vi "LoadFiles.vi"   [LabVIEW 2014]
uses:
  Common Code/Change Detect Int.vi
  Robot Global Data.vi
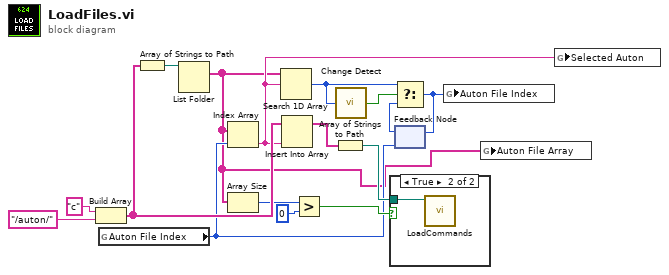
[diagram p0: block diagram]
diagram:
  n1 = Build Array("c", "/auton/") -> (w13:string[])
  n2 = global read "Robot Global Data.vi" "Auton File Index"() -> (w4:i32)
  n3 = Array of Strings to Path(0:w13) -> (2:w14:path)  [unwired: 1 in]
  n4 = List Folder(path=w14) -> (filenames=w1:string[])  [unwired: 3 in, 3 out]
  n5 = Index Array(array=w1, index=w4) -> (element=w2:string)
  n6 = Array Size(array=w1) -> (size(s)=w3:i32)
  n7 = Search 1D Array(1D array=w1, element=w2) -> (index of element=w7:i32)  [unwired: 1 in]
  n8 = Insert Into Array(array=w13, new element=w2) -> (w12:string[])  [unwired: 1 in]
  n9 = Greater?(x=w3, y=0) -> (0:w9:bool)
  n10 = Array of Strings to Path(0:w12) -> (2:w10:path)  [unwired: 1 in]
  n11 = call-poly "Change Detect.vi"("In"=w7) -> ("Changed?"=w8:bool)
  n12 = case shown="True" w9 {
    tunnel: w10 -> [_ w17]
    frame False {
    }
    frame True {
      n13 = call "LoadCommands.vi"("File"=w17) -> ()  [unwired: 11 in]
    }
  }
  n14 = feedback #1(w4) -> (w5:i32)
  n15 = Select(t=w7, s=w8, f=w5) -> (s? t:f=w6:i32)
  n16 = feedback-in #1(w6) -> ()
  n17 = global write "Robot Global Data.vi" "Auton File Index"(w6) -> ()
  n18 = global write "Robot Global Data.vi" "Auton File Array"(w1) -> ()
  n19 = global write "Robot Global Data.vi" "Selected Auton"(w2) -> ()
